vi "FileWriteTestLinuxRT.vi"() -> ()   [LabVIEW 2017]
uses:
  State.ctl
panel:
  out "Write Iterations":i32
  in  "Iterations":i64=250
  in  "Log File Name":string="FileWriteTest1"
  in  "Files Written Per Iteration":i64=250
  out "Elapsed Time This Iteration (ms)":u32
  out "error out":errorcluster
  in  "Folder Name":string="FileWriteTest1"
  in  "stop":bool
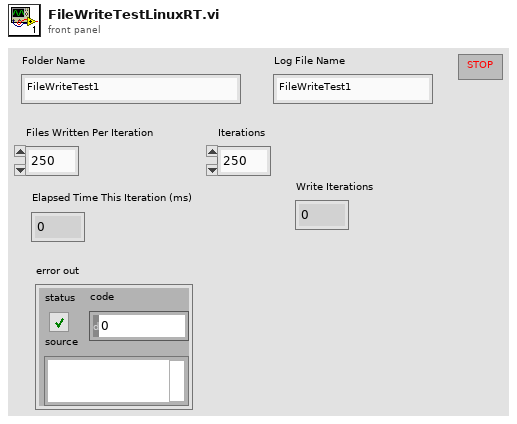
[diagram p1: front panel]
types:
  T1 = typedef "State.ctl" = enum16{"Initialize", "Write", "Log", "Stop"}
  T2 = enum16{"open", "replace", "create", "open or create", "replace or create", "replace or create with confirmation"}
  T3 = enum16{"open", "open or create", "create or replace", "create", "open (read-only)"}
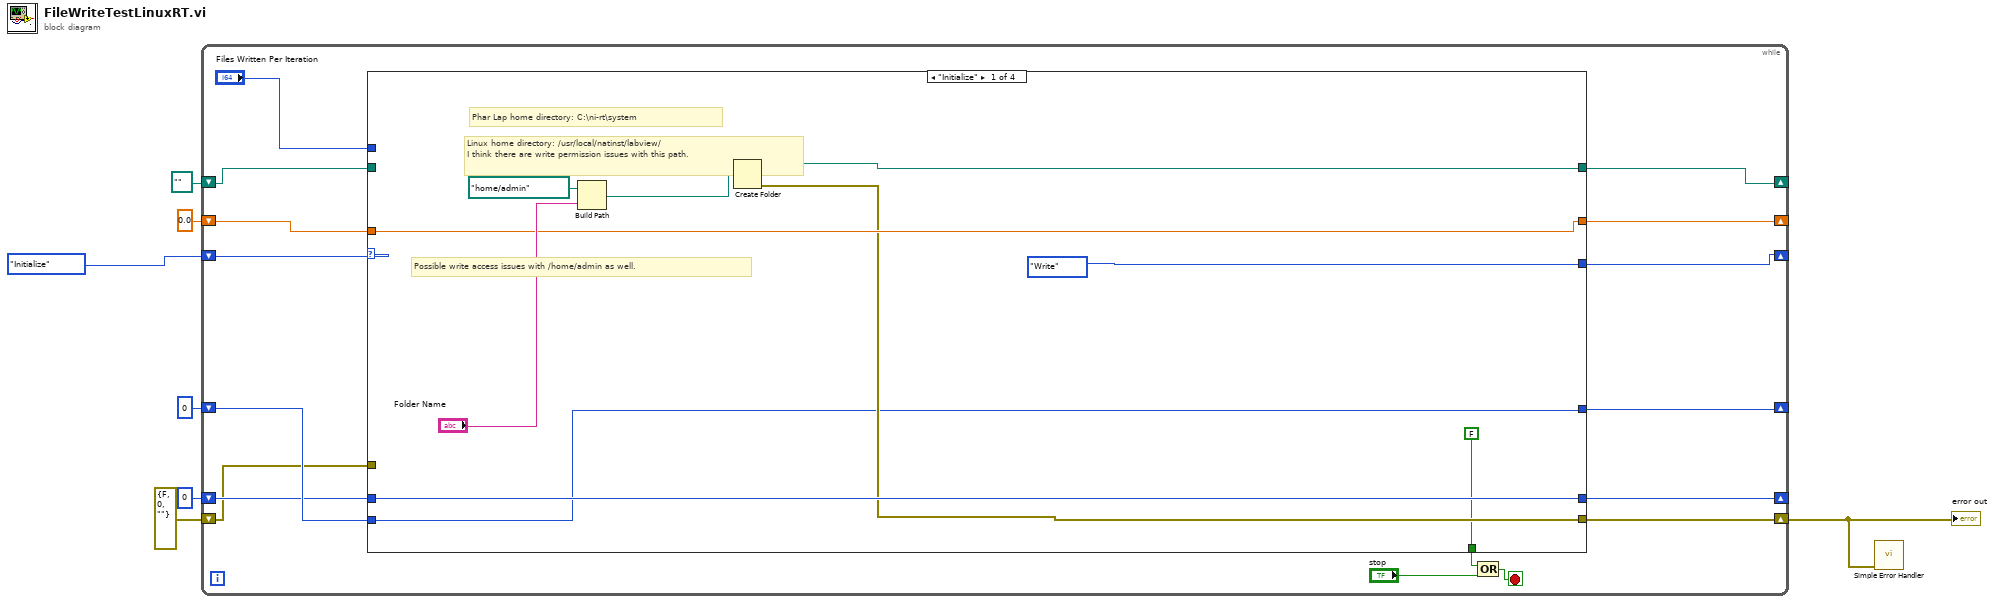
[diagram p0: block diagram]
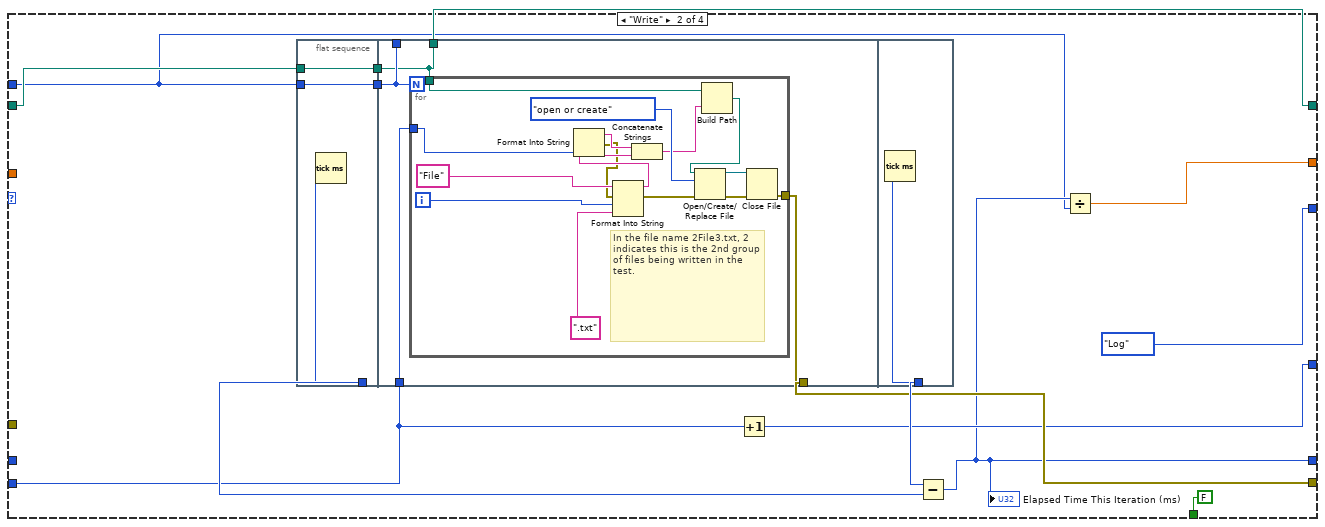
[diagram p2: hidden frame]
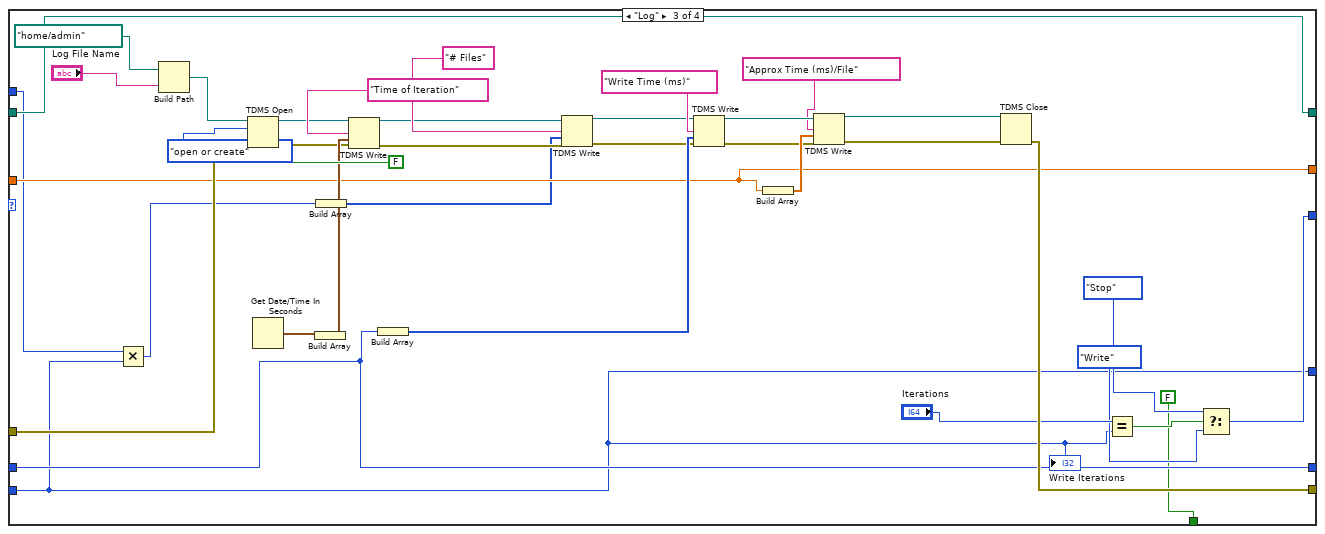
[diagram p3: hidden frame]
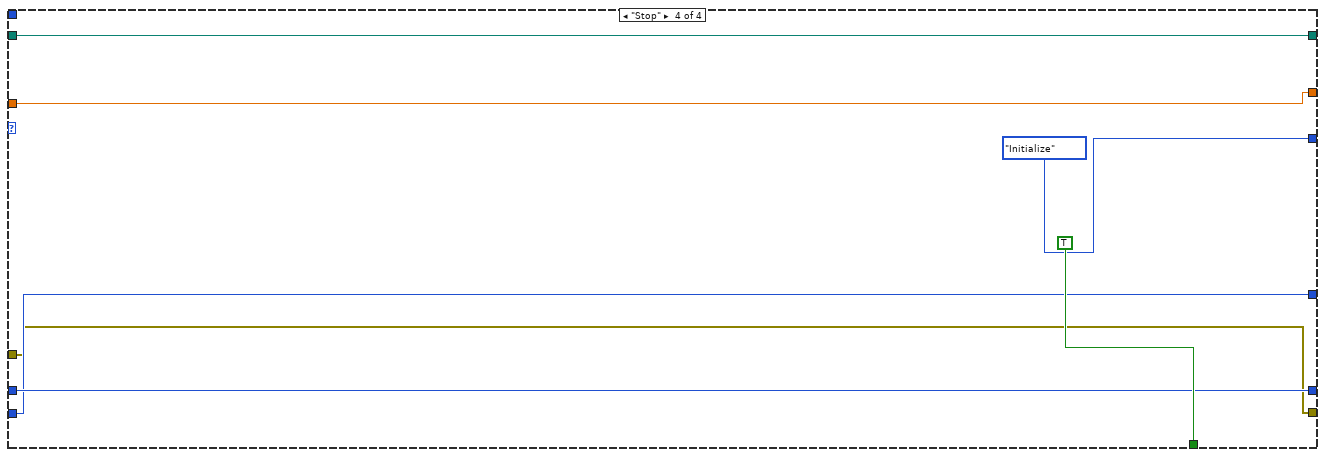
[diagram p4: hidden frame]
diagram:
  n1 = while {
    shift-right: [w11] -> _
    shift-left: State."Initialize" -> [w23]
    shift-right: [w21] -> _
    shift-left: path "" ("created path") -> [w20]
    shift-right: [w19] -> _
    shift-left: u32 0 -> [w15]
    shift-right: [w18] -> w6
    shift-left: errorcluster {"status"=FALSE, "code"=0, "source"=""} ("error out") -> [w12]
    shift-right: [w17] -> _
    shift-left: 0 ("Write Iterations") -> [w16]
    shift-right: [w14] -> _
    shift-left: 0.0 -> [w13]
    stop <- w8 stop-if-true
    n2 = case shown="\"Initialize\"" w23 {
      tunnel: "Files Written Per Iteration" -> [_ w35 w74 _]
      tunnel: [w28 w38 w84 w109] -> w21
      tunnel: w20 -> [_ w40 w84 w109]
      tunnel: [w31 w36 w85 w114] -> w19
      tunnel: [w29 w44 w87 w110] -> w18
      tunnel: [w26 w43 w73 w113] -> w17
      tunnel: w16 -> [w26 w37 w73 w113]
      tunnel: w15 -> [w31 _ w85 w114]
      tunnel: [w32 w42 w86 w112] -> w14
      tunnel: w13 -> [w32 _ w86 w112]
      tunnel: w12 -> [_ _ w93 w110]
      tunnel: [State."Write" State."Log" w76 State."Initialize"] -> w11
      tunnel: [FALSE ("Boolean") FALSE ("Boolean") FALSE ("Boolean") TRUE] -> w10
      frame "Initialize" {
        # "Possible write access issues with /home/admin as well."
        # "Linux home directory: /usr/local/natinst/labview/\nI think there are write permission issues with this path."
        # "Phar Lap home directory: C:\\ni-rt\\system"
        n3 = Build Path(base path=path "/home/admin", name or relative path="Folder Name") -> (appended path=w30:path)
        n4 = Create Folder(path (use dialog)=w30) -> (created path=w28:path, error out=w29:errorcluster)  [unwired: 2 in, 1 out]
      }
      frame "Write" {
        n5 = flat-sequence {
          tunnel: w35 -> [w50]
          tunnel: [w50] -> w47
          tunnel: [w49] -> w45
          tunnel: w40 -> [w48]
          tunnel: [w48] -> w39
          tunnel: w47 -> [w53]
          tunnel: [w54] -> w44
          tunnel: [w53] -> _
          tunnel: w39 -> [w52]
          tunnel: [w52] -> w38
          tunnel: w37 -> [w51]
          tunnel: [w70] -> w46
          frame #0 {
            n6 = Tick Count (ms)() -> (millisecond timer value=w49:u32)
          }
          frame #1 {
            n7 = for {
              N: w53 -> [_]
              tunnel: [w62] -> w54
              tunnel: w52 -> [w61]
              tunnel: w51 -> [w57]
              i -> [w68]
              # "In the file name 2File3.txt, 2 indicates this is the 2nd group of files being written in the test."
              n8 = Format Into String(w57) -> (resulting string=w56:string, error out=w55:errorcluster)  [unwired: 3 in]
              n9 = Format Into String(initial string="File", error in=w55, w68, ".txt") -> (resulting string=w59:string, error out=w66:errorcluster)  [unwired: 1 in]
              n10 = Concatenate Strings(w56, w59) -> (w60:string)
              n11 = Build Path(base path=w61, name or relative path=w60) -> (appended path=w65:path)
              n12 = Open/Create/Replace File(file path (use dialog)=w65, error in=w66, operation (0:open)=T2."open or create") -> (refnum out=w64:refnum<file>, error out=w63:errorcluster)  [unwired: 3 in, 1 out]
              n13 = Close File(refnum=w64, error in=w63) -> (error out=w62:errorcluster)  [unwired: 1 out]
            }
          }
          frame #2 {
            n14 = Tick Count (ms)() -> (millisecond timer value=w70:u32)
          }
        }
        n15 = Increment(x=w37) -> (x+1=w43:i32)
        n16 = Subtract(x=w46, y=w45) -> (x-y=w36:u32)
        "Elapsed Time This Iteration (ms)" <- w36
        n17 = Divide(x=w36, y=w35) -> (x/y=w42:dbl)
      }
      frame "Log" {
        n18 = Multiply(x=w74, y=w73) -> (x*y=w72:i64)
        n19 = Build Path(base path=path "/home/admin", name or relative path="Log File Name") -> (appended path=w82:path)
        n20 = TDMS Open(6:FALSE ("disable buffering (T)"), 8:w93, 10:T3."open or create" ("operation"), 11:w82) -> (0:w92:errorcluster, 3:w105:refnum<k34>)  [unwired: 3 in]
        n21 = Get Date/Time In Seconds() -> (seconds since 1Jan1904=w104:timestamp)
        n22 = Build Array(w104) -> (w103:timestamp[])
        n23 = Build Array(w72) -> (w75:i64[])
        n24 = TDMS Write(0:w105, 7:"Time of Iteration", 9:w103, 11:w92) -> (4:w99:refnum<k34>, 15:w91:errorcluster)  [unwired: 2 in, 2 out]
        n25 = Build Array(w85) -> (w101:u32[])
        n26 = TDMS Write(0:w99, 7:"# Files", 9:w75, 11:w91) -> (4:w98:refnum<k34>, 15:w90:errorcluster)  [unwired: 2 in, 2 out]
        n27 = TDMS Write(0:w98, 7:"Write Time (ms)", 9:w101, 11:w90) -> (4:w97:refnum<k34>, 15:w89:errorcluster)  [unwired: 2 in, 2 out]
        n28 = Build Array(w86) -> (w96:dbl[])
        n29 = TDMS Write(0:w97, 7:"Approx Time (ms)/File", 9:w96, 11:w89) -> (4:w94:refnum<k34>, 15:w88:errorcluster)  [unwired: 2 in, 2 out]
        n30 = TDMS Close(8:w88, 11:w94) -> (0:w87:errorcluster)  [unwired: 1 out]
        n31 = Equal?(x="Iterations", y=w73) -> (x = y?=w80:bool)
        n32 = Select(t=State."Stop", s=w80, f=State."Write") -> (s? t:f=w76:T1)
        "Write Iterations" <- w73
      }
      frame "Stop" {
      }
    }
    n33 = Compound Arithmetic op=OR(w10, "stop") -> (w8:bool)
  }
  "error out" <- w6
  n34 = call <vilib>:"Simple Error Handler.vi"("error in (no error)"=w6) -> ()  [unwired: 4 in, 5 out]
